vi "Generate Date Time Stamp (SubVI).vi"(10 "Experiment Mode":T1, 11 "Movie File Path":path=path "E:/Rawdata/72F11-Gal4xUAS-CsChrimson_20180513_192634.dbde") -> (3 "Date Time String":string)   [LabVIEW 2020]
uses:
  Controls (HOST)/Experiment Mode.ctl
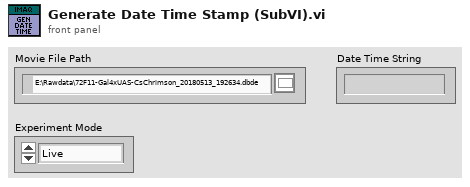
[diagram p1: front panel]
types:
  T1 = typedef "Experiment Mode.ctl" = enum16{"Live", "Replay"}
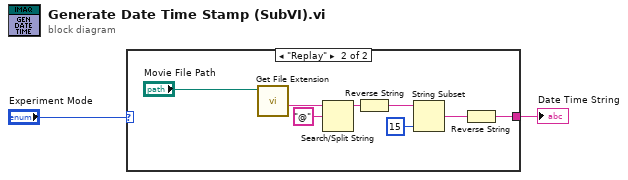
[diagram p0: block diagram]
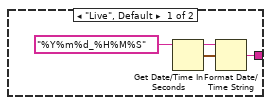
[diagram p2: hidden frame]
diagram:
  n1 = case shown="\"Replay\"" "Experiment Mode" {
    tunnel: [w3 w7] -> w1
    frame "Live", Default {
      n2 = Get Date/Time In Seconds() -> (seconds since 1Jan1904=w4:timestamp)
      n3 = Format Date/Time String(time format string (%c)="%Y%m%d_%H%M%S", seconds (now)=w4) -> (date/time string=w3:string)  [unwired: 1 in]
    }
    frame "Replay" {
      n4 = call <vilib>:"Get File Extension.vi"("file"="Movie File Path") -> ("filename without extension"=w12:string)  [unwired: 6 in, 4 out]
      n5 = Search/Split String(string=w12, search string/char (-)="@") -> (substring before match=w11:string)  [unwired: 1 in, 2 out]
      n6 = Reverse String(1:w11) -> (0:w10:string)
      n7 = String Subset(string=w10, length (rest)=15 ("length (rest)")) -> (substring=w8:string)  [unwired: 1 in]
      n8 = Reverse String(1:w8) -> (0:w7:string)
    }
  }
  "Date Time String" <- w1
